vi "SetPayloadCluster.vi"(7 "Message":refnum<class "Message.lvclass">, 11 "PayloadCluster":T1 {"MetadataCluster"."AbsoluteTime" format="%<%x %.3X>T"}) -> (5 "Message":refnum<class "Message.lvclass">)   [LabVIEW 2020, in "_Template.lvlib" / "{{Message}}.lvlib" / "Message.lvclass"]
uses:
  Message.lvclass
  Message.lvclass/Message.ctl
  jettl/jettl/LifecycleEnum.ctl
  jettl/jettl/jettl.lvlib
  jettl/jettl/TellOriginEnum.ctl
  jettl/jettl/MetadataCluster.ctl
  PayloadCluster.ctl
  {{Message}}.lvlib
panel:
  # "This front panel should not be manipulated."
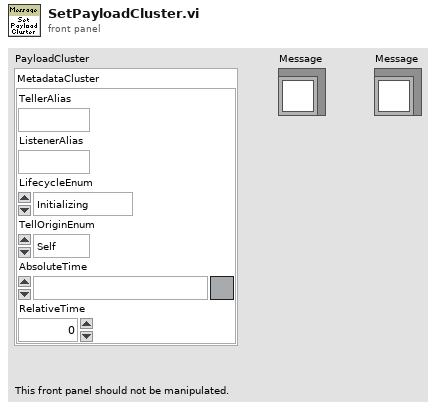
[diagram p1: front panel]
types:
  T1 = typedef "_Template.lvlib/{{Message}}.lvlib/PayloadCluster.ctl" = cluster{"MetadataCluster":T2}
  T2 = typedef "jettl.lvlib/MetadataCluster.ctl" = cluster{"TellerAlias":string, "ListenerAlias":string, "LifecycleEnum":T3, "TellOriginEnum":T4, "AbsoluteTime":timestamp, "RelativeTime":dbl}
  T3 = typedef "jettl.lvlib/LifecycleEnum.ctl" = enum16{"Initializing", "SettingUp", "Starting", "Running", "Stopping", "TearingDown", "Terminated"}
  T4 = typedef "jettl.lvlib/TellOriginEnum.ctl" = enum16{"Self", "Mediator", "Component"}
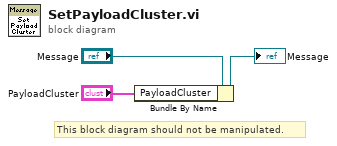
[diagram p0: block diagram]
diagram:
  # "This block diagram should not be manipulated."
  n1 = Bundle By Name(cluster="Message", "PayloadCluster"="PayloadCluster") -> (→"Message":refnum<class "Message.lvclass">)
